vi "CTO_Query.vi"(0 "System no.":i32=1 min=1 max=4 step=1, 2 "TriggerOut to query In":string[](array[string]), 3 "CTO parameter ID":i32[](array[numeric]), 4 "All Triggers?":bool, 5 "error in":errorcluster) -> (15 "Parameter value":string[](array[string]), 16 "TriggerOut to query out":string[](array[string]), 17 "CTO parameter ID out":i32[](array[numeric]), 19 "error out":errorcluster)   [LabVIEW 2020]
doc: "Returns the Trigger Output configuration for the given trigger output line. \n\nC-413: TriggerOut to query can be 1 to 5.\nC-702: TriggerOut to query can be 1 to 8.\nC-843: TriggerOut to query can be 1 to 4 (4-axis card) or 2 (2-axis card).\nC-866: TriggerOut to query can be 1.\nC-867, C-877: Check controller user manual for available output trigger numbers. \nC-884, E-871, E-873, E-874: Check controller user manual for available output trigger numbers. \nE-517, E-518: TriggerOut to query can be 1 to 3.\nE-709: TriggerOut to query can be 1 to 2.\nE-712: TriggerOut to query can be 1 to 7.\nE-725: TriggerOut to query can be 1 to 7.\nE-727: TriggerOut to query can be 1 to 3.\nE-753: TriggerOut to query can be 1.\nE-754: TriggerOut to query can be 1.\nMercury: TriggerOut to query can be 1 to N (N: number of connected axes, if supported by corresponding Mercury firmware).\nMercury_GCS: Check Mercury user manual for available output trigger numbers."
uses:
  Global1.vi
panel:
  # "Returns the Trigger Output configuration for the given trigger output line."
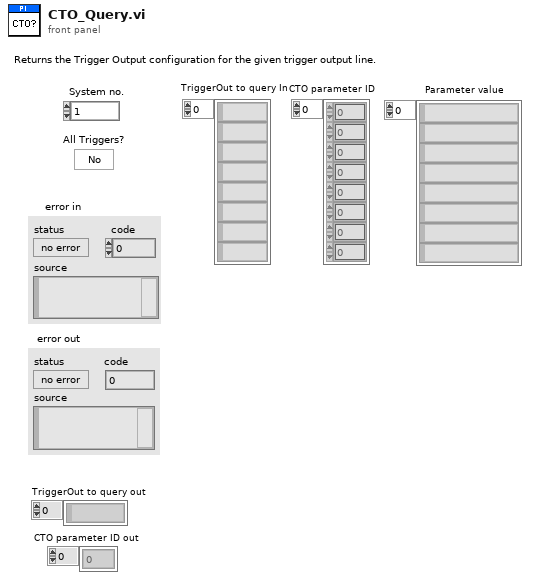
[diagram p1: front panel]
types:
  T1 = typedef "Syntax.ctl" = enum16{"GCS 1.0", "GCS 2.0", "GCS 3.0"}
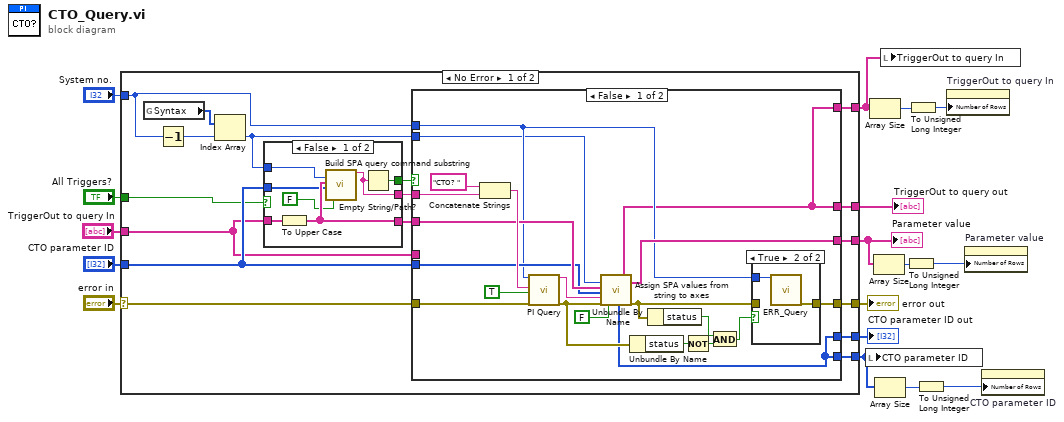
[diagram p0: block diagram]
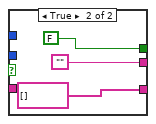
[diagram p2: hidden frame]
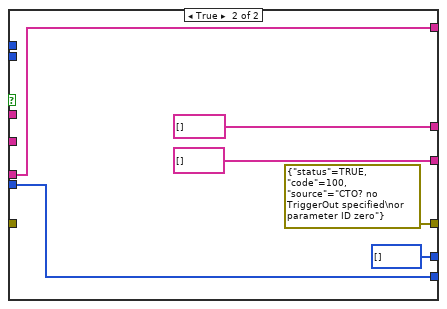
[diagram p4: hidden frame]
diagram:
  n1 = case shown="No Error" "error in" {
    selector: "error in" -> [w24 w79]
    tunnel: "TriggerOut to query In" -> [w19 w76]
    tunnel: "System no." -> [w23 _]
    tunnel: "CTO parameter ID" -> [w32 w75]
    tunnel: [w31 w79] -> w14
    tunnel: "All Triggers?" -> [w29 _]
    tunnel: [w28 string[] [] ("Parameter strings")] -> w7
    tunnel: [w22 string[] [] ("Queried axes out")] -> w11
    tunnel: [w21 i32[] [] ("Parameter no. out")] -> w4
    tunnel: [w18 w75] -> w3
    tunnel: [w20 w76] -> w1
    frame No Error {
      n2 = global read "Global1.vi" "Syntax"() -> (w26:T1[])
      n3 = Decrement(x=w23) -> (x-1=w27:i32)
      n4 = Index Array(array=w26, index=w27) -> (element=w25:T1)
      n5 = case shown="False" w29 {
        tunnel: w19 -> [w41 _]
        tunnel: [w35 "" ("Command substring")] -> w34
        tunnel: [w40 string[] [] ("Designator to query")] -> w33
        tunnel: w32 -> [w39 _]
        tunnel: [w36 FALSE] -> w30
        tunnel: w25 -> [w38 _]
        frame False {
          n6 = To Upper Case(1:w41) -> (0:w40:string[])
          n7 = call "Build SPA query command substring.vi"("Syntax"=w38, "Axes to query"=w40, "Parameter number"=w39, "Parameter no. format \n(Decimal: FALSE)"=FALSE ("Parameter no. format \n(Decimal: FALSE)")) -> ("Command substring"=w35:string)  [unwired: 3 in, 12 out]
          n8 = Empty String/Path?(string/path=w35) -> (empty?=w36:bool)
        }
        frame True {
        }
      }
      n9 = case shown="False" w30 {
        tunnel: w24 -> [w54 _]
        tunnel: w34 -> [w62 _]
        tunnel: w33 -> [w61 _]
        tunnel: w23 -> [w53 _]
        tunnel: w32 -> [w60 w69]
        tunnel: [w56 errorcluster {"status"=TRUE, "code"=100, "source"="CTO? no TriggerOut specified\nor parameter ID zero"} ("error out")] -> w31
        tunnel: [w55 string[] [] ("Parameter strings")] -> w28
        tunnel: w25 -> [w52 _]
        tunnel: [w46 string[] [] ("Queried axes out")] -> w22
        tunnel: [w45 i32[] [] ("Parameter no. out")] -> w21
        tunnel: [w46 w70] -> w20
        tunnel: w19 -> [_ w70]
        tunnel: [w45 w69] -> w18
        frame False {
          n10 = Concatenate Strings("CTO? ", w62) -> (w63:string)
          n11 = call "PI Query.vi"("System no."=w53, "String to send"=w63, "Attach termination char.?"=TRUE ("Attach Linefeed?"), "error in"=w54) -> ("String read"=w50:string, "error out"=w49:errorcluster)  [unwired: 3 in, 11 out]
          n12 = call "Assign SPA values from string to axes.vi"("Syntax"=w52, "Queried axes"=w61, "Parameter no."=w60, "Input string"=w50, "error in"=w49, "Parameter no. format \n(Decimal: FALSE)"=FALSE ("Parameter no. format \n(Decimal: FALSE)")) -> ("Parameter no. out"=w45:i32[], "Queried axes out"=w46:string[], "Parameter strings"=w55:string[], "error out"=w57:errorcluster)  [unwired: 2 in, 8 out]
          n13 = Unbundle By Name(w49) -> ("status"=w47:bool)
          n14 = Unbundle By Name(w57) -> ("status"=w59:bool)
          n15 = Not(x=w47) -> (.not. x?=w48:bool)
          n16 = And(x=w59, y=w48) -> (x .and. y?=w58:bool)
          n17 = case shown="True" w58 {
            tunnel: w57 -> [w66 _]
            tunnel: [w66 w67] -> w56
            tunnel: w53 -> [_ w68]
            frame False {
            }
            frame True {
              n18 = call "ERR_Query.vi"("System no."=w68) -> ("error out"=w67:errorcluster)  [unwired: 1 in, 17 out]
            }
          }
        }
        frame True {
        }
      }
    }
    frame Error {
    }
  }
  "error out" <- w14
  "Parameter value" <- w7
  "TriggerOut to query out" <- w11
  "CTO parameter ID out" <- w4
  n19 = local write "CTO parameter ID"(w3) -> ()
  n20 = Array Size(array=w1) -> (size(s)=w8:i32)
  n21 = Array Size(array=w7) -> (size(s)=w10:i32)
  n22 = Array Size(array=w3) -> (size(s)=w6:i32)
  n23 = local write "TriggerOut to query In"(w1) -> ()
  n24 = To Unsigned Long Integer(number=w10) -> (unsigned 32bit integer=w9:u32)
  n25 = To Unsigned Long Integer(number=w8) -> (unsigned 32bit integer=w2:u32)
  n26 = To Unsigned Long Integer(number=w6) -> (unsigned 32bit integer=w5:u32)
  n27 = property on="TriggerOut to query In" class="Arr (strict)"("Number of Rows"=w2) -> ()  [unwired: 2 in, 2 out]
  n28 = property on="Parameter value" class="Arr (strict)"("Number of Rows"=w9) -> ()  [unwired: 2 in, 2 out]
  n29 = property on="CTO parameter ID" class="Arr (strict)"("Number of Rows"=w5) -> ()  [unwired: 2 in, 2 out]
